vi "FTW-CodeGen-Prototype.vi"(0 "REPLACED_SQLite Connector":refnum<class "FTW-SQLite-Connector.lvclass">, 2 "REPLACED_SQL Script":string, 5 "ADAPT_Data to Insert":T1(array[cluster]), 7 "REPLACED_Pre-Process SQL":string="BEGIN TRANSACTION;", 9 "REPLACED_Post-Process SQL":string="COMMIT TRANSACTION;", 11 "REPLACED_error in":errorcluster) -> (4 "REPLACED_SQLite Connector out":refnum<class "FTW-SQLite-Connector.lvclass">, 6 "REPLACED_Time to Execute+Compile":dbl format="%.6fsec", 8 "REPLACED_Time to Compile SQL":dbl format="%.6fsec", 15 "REPLACED_error out":errorcluster)   [LabVIEW 2013, in "FTW-SQLite-Insert.xnode"]
uses:
  FTW-SQLite-Insert.xnode
  src/Database/FTW-SQLite-Connector.lvclass
panel:
  # "Inputs"
  # "Outputs"
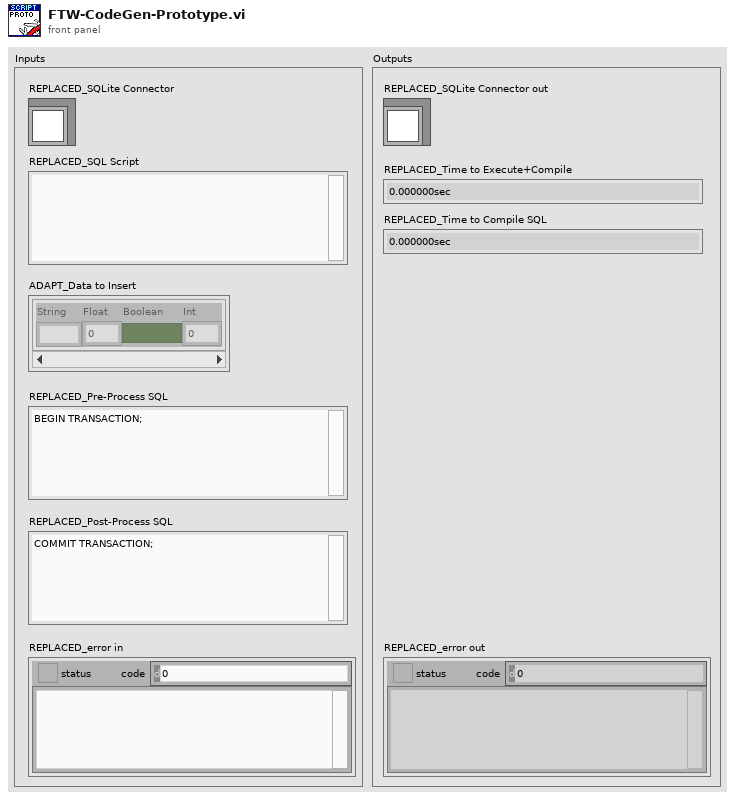
[diagram p1: front panel]
types:
  T1 = cluster{"String":string, "Float":dbl, "Boolean":bool, "Int":i64}[]
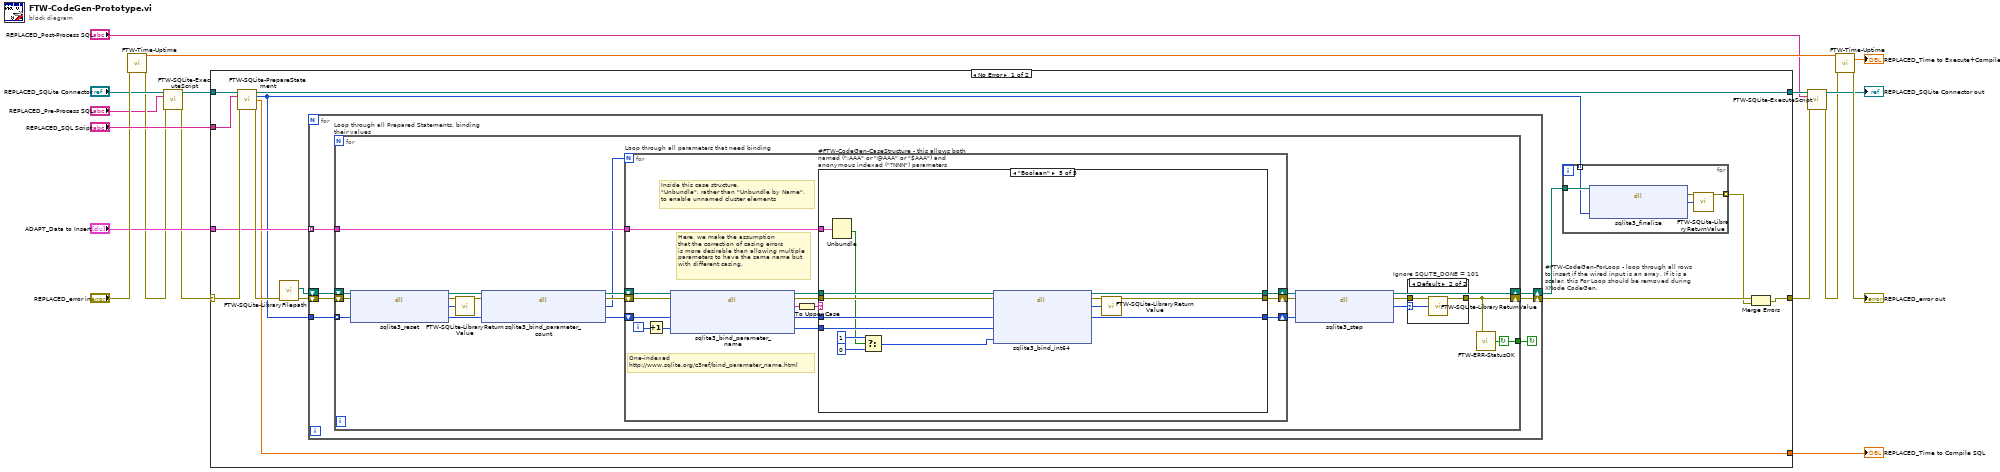
[diagram p0: block diagram]
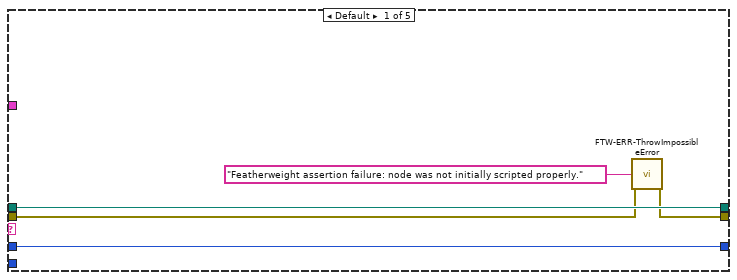
[diagram p3: hidden frame]
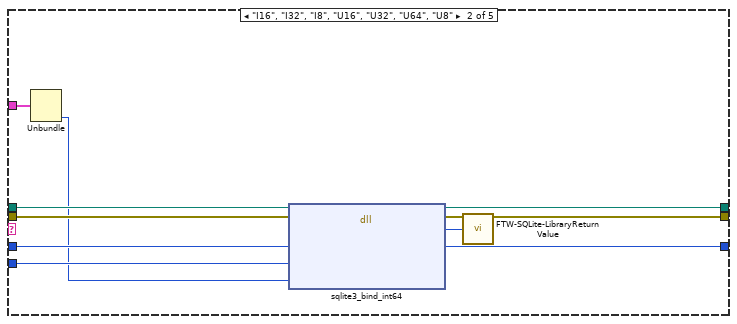
[diagram p4: hidden frame]
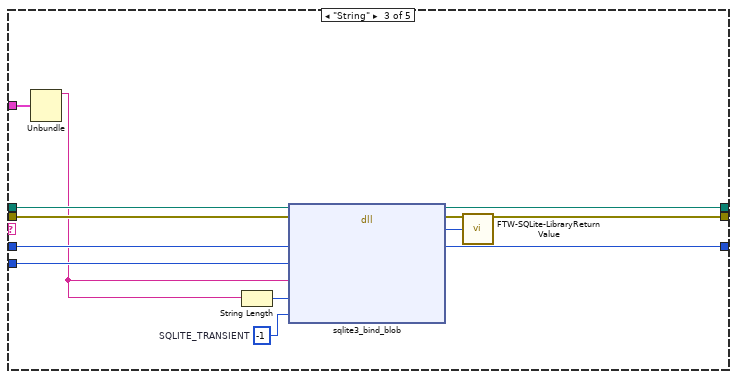
[diagram p5: hidden frame]
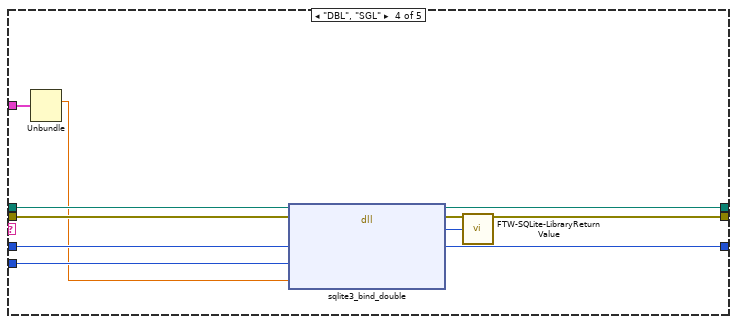
[diagram p6: hidden frame]
diagram:
  n1 = call "FTW-Time-Uptime.vi"("error in"="REPLACED_error in") -> ("Current Uptime"=w14:dbl, "error out"=w8:errorcluster)  [unwired: 12 in, 1 out]
  n2 = call "FTW-SQLite-ExecuteScript.vi"("SQLite Connector"="REPLACED_SQLite Connector", "SQL Script"="REPLACED_Pre-Process SQL", "error in"=w8) -> ("SQLite Connector out"=w9:refnum<class "FTW-SQLite-Connector.lvclass">, "error out"=w7:errorcluster)  [unwired: 9 in, 2 out]
  n3 = case shown="No Error" w7 {
    selector: w7 -> [w30 w138]
    tunnel: w9 -> [w31 w139]
    tunnel: [w29 w139] -> w4
    tunnel: "REPLACED_SQL Script" -> [w28 _]
    tunnel: [w20 w138] -> w2
    tunnel: "ADAPT_Data to Insert" -> [w24 _]
    tunnel: [w23 _] -> w12
    frame No Error {
      n4 = call "FTW-SQLite-PrepareStatement.vi"("SQLite Connector"=w31, "SQL Statement"=w28, "error in"=w30) -> ("SQLite Connector out"=w29:refnum<class "FTW-SQLite-Connector.lvclass">, "Prepared Statements"=w18:i64[], "Time to Compile SQL"=w23:dbl, "error out"=w27:errorcluster)  [unwired: 9 in]
      n5 = call "FTW-SQLite-LibraryFilepath.vi"("error in"=w27) -> ("error out"=w26:errorcluster, "SQLite Library Filepath"=w25:path)  [unwired: 8 in, 1 out]
      n6 = for "#FTW-CodeGen-ForLoop - loop through all rows to insert if the wired input is an array. If it is a scalar, this For Loop should be removed during XNode CodeGen." {
        tunnel: w18 -> [w40]
        shift-right: [w39] -> w21
        shift-left: w26 -> [w41]
        tunnel: w24 -> [w43] mode=indexing
        shift-right: [w38] -> w22
        shift-left: w25 -> [w42]
        stop <- w37 continue-if-true
        n7 = for "Loop through all Prepared Statements, binding their values" {
          shift-right: [w61] -> w38
          shift-left: w42 -> [w52]
          shift-right: [w59] -> w39
          shift-left: w41 -> [w51]
          tunnel: w43 -> [w58]
          tunnel: w40 -> [w50] mode=indexing
          tunnel: [w44] -> w37
          stop <- w44 continue-if-true
          n8 = dll-call lib="?" fn="sqlite3_reset"(path in=w52, error in=w51, "Prepared Statement Pointer"=w50) -> (path out=w45:path, error out=w49:errorcluster, "Return Value"=w46:i32, "Prepared Statement Pointer"=w47:i64)  [unwired: 1 in]
          n9 = call "FTW-SQLite-LibraryReturnValue.vi"("error in"=w49, "Return Value"=w46) -> ("error out"=w48:errorcluster)  [unwired: 13 in]
          n10 = dll-call lib="?" fn="sqlite3_bind_parameter_count"(path in=w45, error in=w48, "Prepared Statement Pointer"=w47) -> (path out=w57:path, error out=w56:errorcluster, "Num Parameters to Bind"=w54:i32, "Prepared Statement Pointer"=w55:i64)  [unwired: 1 in]
          n11 = for "Loop through all parameters that need binding" {
            N: w54 -> [_]
            shift-right: [w83] -> w64
            shift-left: w57 -> [w79]
            shift-right: [w81] -> w63
            shift-left: w56 -> [w77]
            shift-right: [w82] -> w62
            shift-left: w55 -> [w75]
            tunnel: w58 -> [w80]
            i -> [w72]
            # "Inside this case structure,\n\"Unbundle\", rather than \"Unbundle by Name\",\nto enable unnamed cluster elements"
            # "Here, we make the assumption\nthat the correction of casing errors\nis more desirable than allowing multiple\nparameters to have the same name but\nwith different casing."
            # "One-indexed\nhttp://www.sqlite.org/c3ref/bind_parameter_name.html"
            n12 = Increment(x=w72) -> (x+1=w69:i32)
            n13 = dll-call lib="?" fn="sqlite3_bind_parameter_name"(path in=w79, error in=w77, "Prepared Statement Pointer"=w75, "Parameter Index"=w69) -> (path out=w78:path, error out=w76:errorcluster, "Parameter Name"=w73:string, "Prepared Statement Pointer"=w74:i64, "Parameter Index"=w71:i32)  [unwired: 1 in]
            n14 = To Upper Case(1:w73) -> (0:w70:string)
            n15 = case "#FTW-CodeGen-CaseStructure - this allows both named (\":AAA\" or \"@AAA\" or \"$AAA\") and anonymous indexed (\"?NNN\") parameters" shown="\"Boolean\"" w70 {
              tunnel: w78 -> [w88 w97 w110 w121 w135]
              tunnel: w76 -> [w86 w96 w109 w120 w134]
              tunnel: w74 -> [w87 w95 w108 w119 w133]
              tunnel: [w88 w99 w112 w123 w137] -> w83
              tunnel: [w87 w98 w111 w122 w136] -> w82
              tunnel: [w85 w91 w104 w115 w129] -> w81
              tunnel: w80 -> [_ w93 w106 w117 w131]
              tunnel: w71 -> [_ w94 w107 w118 w132]
              frame Default {
                n16 = call "FTW-ERR-ThrowImpossibleError.vi"("Reason this error should never happen"="Featherweight assertion failure: node was not initially scripted properly.", "error in"=w86) -> ("error out"=w85:errorcluster)  [unwired: 13 in]
              }
              frame "I16", "I32", "I8", "U16", "U32", "U64", "U8" {
                n17 = Unbundle(w93) -> ("Int"=w89:i64)  [unwired: 3 out]
                n18 = dll-call lib="?" fn="sqlite3_bind_int64"(path in=w97, error in=w96, "Prepared Statement Pointer"=w95, "Parameter Index"=w94, "I64 Value"=w89) -> (path out=w99:path, error out=w92:errorcluster, "Return Value"=w90:i32, "Prepared Statement Pointer"=w98:i64)  [unwired: 3 in]
                n19 = call "FTW-SQLite-LibraryReturnValue.vi"("error in"=w92, "Return Value"=w90) -> ("error out"=w91:errorcluster)  [unwired: 13 in]
              }
              frame "String" {
                w101 = i64 -1  # SQLITE_TRANSIENT
                n20 = Unbundle(w106) -> ("String"=w100:string)  [unwired: 3 out]
                n21 = String Length(string=w100) -> (length=w102:i32)
                n22 = dll-call lib="?" fn="sqlite3_bind_blob"(path in=w110, error in=w109, "Prepared Statement Pointer"=w108, "Parameter Index"=w107, "BLOB Value"=w100, "BLOB Size (bytes)"=w102, "BLOB dtor function"=w101) -> (path out=w112:path, error out=w105:errorcluster, "Return Value"=w103:i32, "Prepared Statement Pointer"=w111:i64)  [unwired: 5 in]
                n23 = call "FTW-SQLite-LibraryReturnValue.vi"("error in"=w105, "Return Value"=w103) -> ("error out"=w104:errorcluster)  [unwired: 13 in]
              }
              frame "DBL", "SGL" {
                n24 = Unbundle(w117) -> ("Float"=w113:dbl)  [unwired: 3 out]
                n25 = dll-call lib="?" fn="sqlite3_bind_double"(path in=w121, error in=w120, "Prepared Statement Pointer"=w119, "Parameter Index"=w118, "DBL Value"=w113) -> (path out=w123:path, error out=w116:errorcluster, "Return Value"=w114:i32, "Prepared Statement Pointer"=w122:i64)  [unwired: 3 in]
                n26 = call "FTW-SQLite-LibraryReturnValue.vi"("error in"=w116, "Return Value"=w114) -> ("error out"=w115:errorcluster)  [unwired: 13 in]
              }
              frame "Boolean" {
                n27 = Unbundle(w131) -> ("Boolean"=w124:bool)  [unwired: 3 out]
                n28 = Select(t=i64 1, s=w124, f=i64 0) -> (s? t:f=w127:i64)
                n29 = dll-call lib="?" fn="sqlite3_bind_int64"(path in=w135, error in=w134, "Prepared Statement Pointer"=w133, "Parameter Index"=w132, "I64 Value"=w127) -> (path out=w137:path, error out=w130:errorcluster, "Return Value"=w128:i32, "Prepared Statement Pointer"=w136:i64)  [unwired: 3 in]
                n30 = call "FTW-SQLite-LibraryReturnValue.vi"("error in"=w130, "Return Value"=w128) -> ("error out"=w129:errorcluster)  [unwired: 13 in]
              }
            }
          }
          n31 = dll-call lib="?" fn="sqlite3_step"(path in=w64, error in=w63, "Prepared Statement Pointer"=w62) -> (path out=w61:path, error out=w60:errorcluster, "Return Value"=w53:i32)  [unwired: 2 in]
          n32 = case "Ignore SQLITE_DONE = 101" shown="Default" w53 {
            selector: w53 -> [_ w66]
            tunnel: w60 -> [w65 w68]
            tunnel: [w65 w67] -> w59
            frame 101 {
            }
            frame Default {
              n33 = call "FTW-SQLite-LibraryReturnValue.vi"("error in"=w68, "Return Value"=w66) -> ("error out"=w67:errorcluster)  [unwired: 13 in]
            }
          }
          n34 = call "FTW-ERR-StatusOK.vi"("error to check"=w59) -> ("Status OK?"=w44:bool)
        }
      }
      n35 = for {
        tunnel: w22 -> [w34]
        tunnel: [w33] -> w19 mode=indexing
        tunnel: w18 -> [w32] mode=indexing
        n36 = dll-call lib="?" fn="sqlite3_finalize"(path in=w34, "Prepared Statement Pointer"=w32) -> (error out=w36:errorcluster, "Return Value"=w35:i32)  [unwired: 3 in, 1 out]
        n37 = call "FTW-SQLite-LibraryReturnValue.vi"("error in"=w36, "Return Value"=w35) -> ("error out"=w33:errorcluster)  [unwired: 13 in]
      }
      n38 = Merge Errors(w21, w19) -> (w20:errorcluster)
    }
    frame Error {
    }
  }
  "REPLACED_Time to Compile SQL" <- w12
  n39 = call "FTW-SQLite-ExecuteScript.vi"("SQLite Connector"=w4, "SQL Script"="REPLACED_Post-Process SQL", "error in"=w2) -> ("SQLite Connector out"=→"REPLACED_SQLite Connector out":refnum<class "FTW-SQLite-Connector.lvclass">, "error out"=w3:errorcluster)  [unwired: 9 in, 2 out]
  n40 = call "FTW-Time-Uptime.vi"("Previous Uptime"=w14, "error in"=w3) -> ("Elapsed Time"=→"REPLACED_Time to Execute+Compile":dbl, "error out"=→"REPLACED_error out":errorcluster)  [unwired: 11 in, 1 out]
